vi "global.vi"() -> ()   [LabVIEW 2015]
panel:
  out "OptionOK":bool
  out "ChildNo":u32
  out "DeviceNo":u32
  in  "gMaxFileName":i32=256
  in  "PDC_MAX_LUTLIST_NUMBER":i32=4096
  in  "PDC_MAX_PARTITION":i32=128
  in  "PDC_MAX_LIST_NUMBER":i32=256
  in  "gMaxDeviceName":i32=256
  in  "PDC_MAX_DEVICE":i32=64
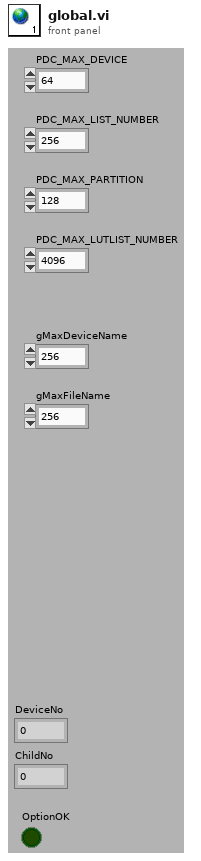
[diagram p1: front panel]
diagram:
